vi "Check File Path.vi"(10 "check if path exists? (F)":bool, 11 "path":path) -> (2 "path exists?":bool, 3 "valid path?":bool)   [LabVIEW 2010, in "NI_SE_Front Panel Layout.lvlib"]
uses:
  NI_SE_Front Panel Layout.lvlib
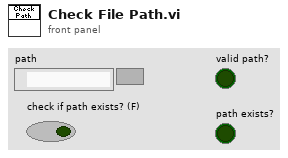
[diagram p1: front panel]
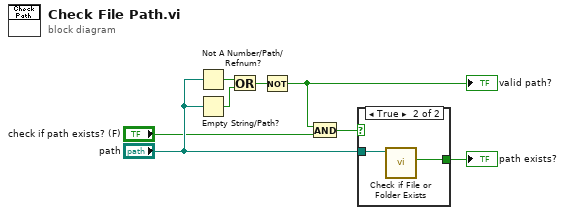
[diagram p0: block diagram]
diagram:
  n1 = Not A Number/Path/Refnum?(number/path/refnum="path") -> (NaN/Path/Refnum?=w8:bool)
  n2 = Empty String/Path?(string/path="path") -> (empty?=w7:bool)
  n3 = Or(x=w8, y=w7) -> (x .or. y?=w6:bool)
  n4 = Not(x=w6) -> (.not. x?=w3:bool)
  "valid path?" <- w3
  n5 = And(x=w3, y="check if path exists? (F)") -> (x .and. y?=w2:bool)
  n6 = case shown="True" w2 {
    tunnel: "path" -> [_ w10]
    tunnel: [_ w9] -> w4
    frame False {
    }
    frame True {
      n7 = call <vilib>:"Check if File or Folder Exists.vi"("path"=w10) -> ("file or folder exists?"=w9:bool)  [unwired: 8 in, 2 out]
    }
  }
  "path exists?" <- w4
